vi "Select Random Solutions.vi"(10 "Population":T1[](array[typedef]), 11 "Tournament Size":i32) -> (3 "Selected Solutions":T1[](array[typedef]))   [LabVIEW 2013, in "GA.lvclass"]
uses:
  GA.lvclass
  Controls/Solution_GA.ctl
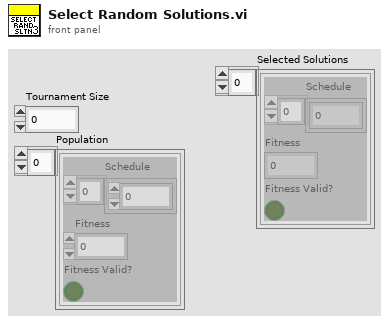
[diagram p1: front panel]
types:
  T1 = typedef "Solution_GA.ctl" = cluster{"Schedule":u16[], "Fitness":u16, "Fitness Valid?":bool}
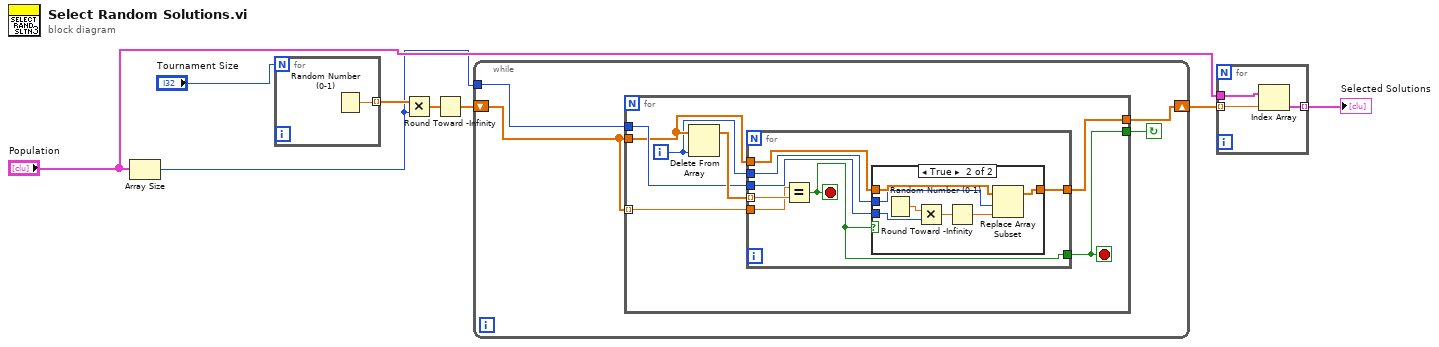
[diagram p0: block diagram]
diagram:
  n1 = Array Size(array="Population") -> (size(s)=w4:i32)
  n2 = for {
    N: "Tournament Size" -> [_]
    tunnel: [w9] -> w6 mode=indexing
    n3 = Random Number (0-1)() -> (number: 0 to 1=w9:dbl)
  }
  n4 = Multiply(x=w6, y=w4) -> (x*y=w5:dbl[])
  n5 = Round Toward -Infinity(1:w5) -> (0:w3:dbl[])
  n6 = while {
    tunnel: w4 -> [w13]
    shift-right: [w12] -> w2
    shift-left: w3 -> [w11]
    stop <- w10 continue-if-true
    n7 = for {
      tunnel: w11 -> [w19] mode=indexing
      tunnel: w11 -> [w17]
      tunnel: w13 -> [w18]
      tunnel: [w15] -> w12
      tunnel: [w14] -> w10
      i -> [w16]
      stop <- w14 stop-if-true
      n8 = Delete From Array(array=w17, index=w16) -> (array with subset deleted=w20:dbl[])  [unwired: 1 in, 1 out]
      n9 = for {
        tunnel: w20 -> [w27] mode=indexing
        tunnel: w19 -> [w26]
        tunnel: w18 -> [w25]
        tunnel: w17 -> [w24]
        tunnel: w16 -> [w23]
        tunnel: [w22] -> w15
        tunnel: [w21] -> w14
        stop <- w21 stop-if-true
        n10 = Equal?(x=w26, y=w27) -> (x = y?=w21:bool)
        n11 = case shown="True" w21 {
          tunnel: w25 -> [_ w34]
          tunnel: w24 -> [w28 w32]
          tunnel: w23 -> [_ w31]
          tunnel: [w28 w29] -> w22
          frame False {
          }
          frame True {
            n12 = Random Number (0-1)() -> (number: 0 to 1=w35:dbl)
            n13 = Multiply(x=w35, y=w34) -> (x*y=w33:dbl)
            n14 = Round Toward -Infinity(1:w33) -> (0:w30:dbl)
            n15 = Replace Array Subset(array=w32, new element=w30, index=w31) -> (w29:dbl[])
          }
        }
      }
    }
  }
  n16 = for {
    tunnel: "Population" -> [w38]
    tunnel: w2 -> [w37] mode=indexing
    tunnel: [w36] -> w1 mode=indexing
    n17 = Index Array(array=w38, index=w37) -> (element=w36:T1)
  }
  "Selected Solutions" <- w1
